vi "tachometer.vi"() -> ()   [LabVIEW 2019]
uses:
  <vilib>/myRIO/Instrument Drivers/Onboard IO/DI Block/typedefs/DI Block Reference.ctl
  <vilib>/myRIO/Common/Instrument Driver Framework/Utilities/typedefs/myRIO Generic Hardware Reference.ctl
  <vilib>/myRIO/Common/Instrument Driver Framework/Utilities/typedefs/Hardware Version Enum.ctl
  <vilib>/myRIO/Common/Instrument Driver Framework/Utilities/typedefs/myRIO v1.0 Reference.ctl
  <vilib>/myRIO/Common/Instrument Driver Framework/Utilities/typedefs/Generic FPGA Reference.ctl
  <vilib>/myRIO/Common/Instrument Driver Framework/myRIO v1.0/DI Block/typedefs/DI Block Channels List.ctl
  <vilib>/myRIO/Common/Instrument Driver Framework/myRIO v1.0/DI Block/typedefs/DI Block Channels Enum.ctl
  <vilib>/userdefined/High Color/nirio_resource_hc.ctl
  <vilib>/myRIO/Common/Instrument Driver Framework/myRIO v1.0/DI Block/vis/myRIO v1.1 Open Throughput DI (N Samples).vi
  <vilib>/myRIO/Common/Instrument Driver Framework/Utilities/vis/Validate Channels.vi
  <vilib>/myRIO/Common/Instrument Driver Framework/myRIO v1.0/DI Block/vis/myRIO v1.0 Close DI Block.vi
  <vilib>/myRIO/Common/Instrument Driver Framework/myRIO v1.0/DI Block/vis/myRIO v1.0 Unreserve DI Block.vi
  <vilib>/myRIO/Common/Instrument Driver Framework/myRIO v1.0/Resource Manager/vis/myRIO v1.0 Unreserve Channel List.vi
  <vilib>/myRIO/Common/Instrument Driver Framework/myRIO v1.0/DI Block/vis/myRIO v1.0 Build MUX Configuration DI Block.vi
  <vilib>/myRIO/Common/Instrument Driver Framework/myRIO v1.0/Resource Manager/vis/myRIO v1.0 Unreserve Channel.vi
  <vilib>/myRIO/Common/Instrument Driver Framework/myRIO v1.0/Resource Manager/vis/myRIO v1.0 Build Mutex Name.vi
  <vilib>/Utility/VariantDataType/GetNumericInfo.vi
  <vilib>/Utility/error.llb/Error Cluster From Error Code.vi
  <vilib>/myRIO/Common/Instrument Driver Framework/myRIO v1.0/myRIO v1.1 Open Throughput.vi
  <vilib>/myRIO/Common/Instrument Driver Framework/myRIO v1.0/DI Block/vis/myRIO v1.0 Reserve DI Block.vi
  <vilib>/myRIO/Common/Instrument Driver Framework/myRIO v1.0/myRIO v1.0 Close.vi
  <vilib>/myRIO/Common/Instrument Driver Framework/myRIO v1.0/DI Block/vis/myRIO v1.0 DI Block Read.vi
  <vilib>/myRIO/Common/Instrument Driver Framework/Utilities/vis/Configuration Manager.vi
  <vilib>/myRIO/Common/Instrument Driver Framework/Utilities/vis/IO Manager.vi
  <vilib>/myRIO/Instrument Drivers/Onboard IO/DI Block/vis/myRIO DI N Samples Open.xnode
  <vilib>/myRIO/Instrument Drivers/Onboard IO/DI Block/DI Block.lvlib
panel:
  out "Czas":u32(graph)
  out "size":i32
  out "Waveform Chart":i16[](graph)
  in  "stop":bool
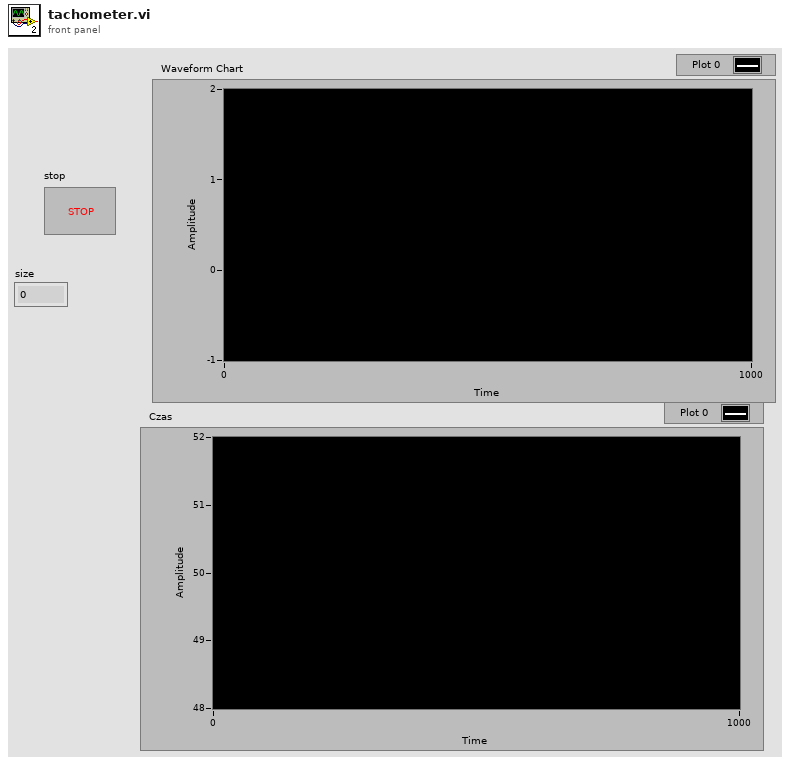
[diagram p1: front panel]
types:
  T1 = typedef "DI Block.lvlib/DI Block Reference.ctl" = cluster{"myRIO Reference":T2, "DI (N Samples) Channels List":T6}
  T2 = typedef "myRIO Generic Hardware Reference.ctl" = cluster{"myRIO Model":T3, "myRIO Hardware Reference":T4}
  T3 = typedef "Hardware Version Enum.ctl" = enum16{"Unknown", "myRIO-1900", "myRIO-1950", "roboRIO", "NI ELVIS RIO CM", "ELVIS III"}
  T4 = typedef "myRIO v1.0 Reference.ctl" = cluster{"Generic FPGA Reference":T5, "Allow multiple opens":bool}
  T5 = typedef "Generic FPGA Reference.ctl" = refnum<k20>
  T6 = typedef "DI Block Channels List.ctl" = T7[]
  T7 = typedef "DI Block Channels Enum.ctl" = enum16{"Not Connected", "A/DI0 (N Samples)", "A/DI1 (N Samples)", "A/DI2 (N Samples)", "A/DI3 (N Samples)", "A/DI4 (N Samples)", "A/DI5 (N Samples)", "A/DI6 (N Samples)", "A/DI7 (N Samples)", "A/DI8 (N Samples)", "A/DI9 (N Samples)", "A/DI10 (N Samples)", "A/DI11 (N Samples)", "A/DI12 (N Samples)", "A/DI13 (N Samples)", "A/DI14 (N Samples)", "A/DI15 (N Samples)", "A/DI16 (N Samples)", "A/DI17 (N Samples)", "A/DI18 (N Samples)", "A/DI19 (N Samples)", "B/DI0 (N Samples)", "B/DI1 (N Samples)", "B/DI2 (N Samples)", "B/DI3 (N Samples)", "B/DI4 (N Samples)", "B/DI5 (N Samples)", "B/DI6 (N Samples)", "B/DI7 (N Samples)", "B/DI8 (N Samples)", "B/DI9 (N Samples)", "B/DI10 (N Samples)", "B/DI11 (N Samples)", "B/DI12 (N Samples)", "B/DI13 (N Samples)", "B/DI14 (N Samples)", "B/DI15 (N Samples)", "B/DI16 (N Samples)", "B/DI17 (N Samples)", "B/DI18 (N Samples)", "B/DI19 (N Samples)"}
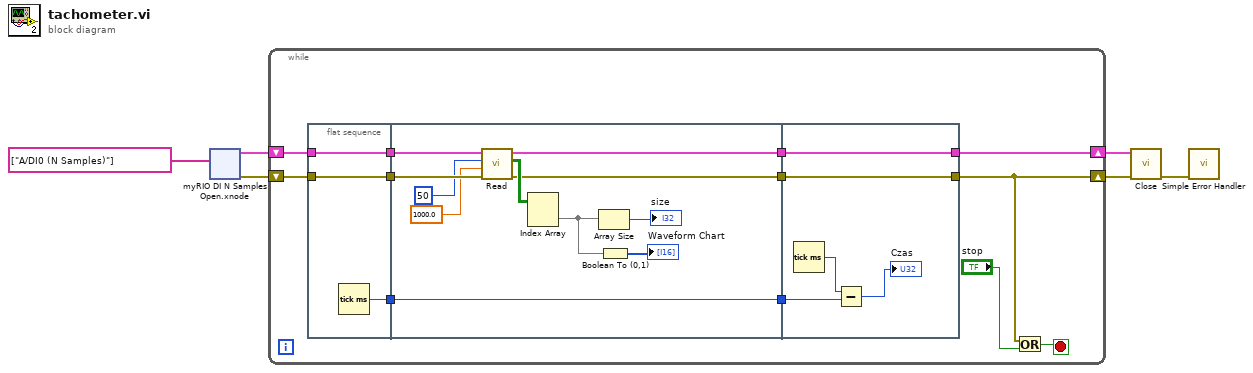
[diagram p0: block diagram]
diagram:
  n1 = xnode "myRIO DI N Samples Open.xnode"("Channel Names"=tag[] ["A/DI0 (N Samples)"]) -> ("error out"=w5:errorcluster, "DI (N Samples) Ref Out"=w6:T1)  [unwired: 2 in]
  n2 = while {
    shift-right: [w16] -> w3
    shift-left: w6 -> [w18]
    shift-right: [w14] -> w4
    shift-left: w5 -> [w17]
    stop <- w15 stop-if-true
    n3 = flat-sequence {
      tunnel: w17 -> [w20]
      tunnel: w18 -> [w21]
      tunnel: [w21] -> w12
      tunnel: [w20] -> w11
      tunnel: [w19] -> w8
      tunnel: w12 -> [w30]
      tunnel: w11 -> [w29]
      tunnel: [w25] -> w10
      tunnel: [w31] -> w9
      tunnel: w8 -> [w31]
      tunnel: [w24] -> w7
      tunnel: [w36] -> w14
      tunnel: [w37] -> w16
      tunnel: w10 -> [w37]
      tunnel: w9 -> [w35]
      tunnel: w7 -> [w36]
      frame #0 {
        n4 = Tick Count (ms)() -> (millisecond timer value=w19:u32)
      }
      frame #1 {
        n5 = call <vilib>:"Read.vi"("error in (no error)"=w29, "Sample Rate [Hz]"=1000.0, "Number of Samples"=u32 50, "DI (N Samples) Ref In"=w30) -> ("error out"=w24:errorcluster, "Values"=w26:bool[][], "DI (N Samples) Ref Out"=w25:T1)  [unwired: 5 in]
        n6 = Index Array(array=w26) -> (element=w23:bool[])  [unwired: 2 in]
        n7 = Array Size(array=w23) -> (size(s)=→"size":i32)
        n8 = Boolean To (0,1)(Boolean=w23) -> (0, 1=→"Waveform Chart":i16[])
      }
      frame #2 {
        n9 = Tick Count (ms)() -> (millisecond timer value=w34:u32)
        n10 = Subtract(x=w34, y=w35) -> (x-y=→"Czas":u32)
      }
    }
    n11 = Or(x=w14, y="stop") -> (x .or. y?=w15:bool)
  }
  n12 = call <vilib>:"Close.vi"("error in (no error)"=w4, "DI (N Samples) Ref In"=w3) -> ("error out"=w2:errorcluster)  [unwired: 9 in]
  n13 = call <vilib>:"Simple Error Handler.vi"("error in (no error)"=w2) -> ()  [unwired: 4 in, 5 out]
